vi "Write device.vi"(8 "error in (no error)":errorcluster, 10 "device":string, 11 "Update Ctl Device Setpoint MSG in":refnum<class "Update Ctl Device Setpoint MSG.lvclass">) -> (0 "error out":errorcluster, 3 "Update Ctl Device Setpoint MSG out":refnum<class "Update Ctl Device Setpoint MSG.lvclass">)   [LabVIEW 2016, in "Controller.lvlib" / "Update Ctl Device Setpoint MSG.lvclass"]
uses:
  Update Ctl Device Setpoint MSG.lvclass
  Update Ctl Device Setpoint MSG.lvclass/Update Ctl Device Setpoint MSG.ctl
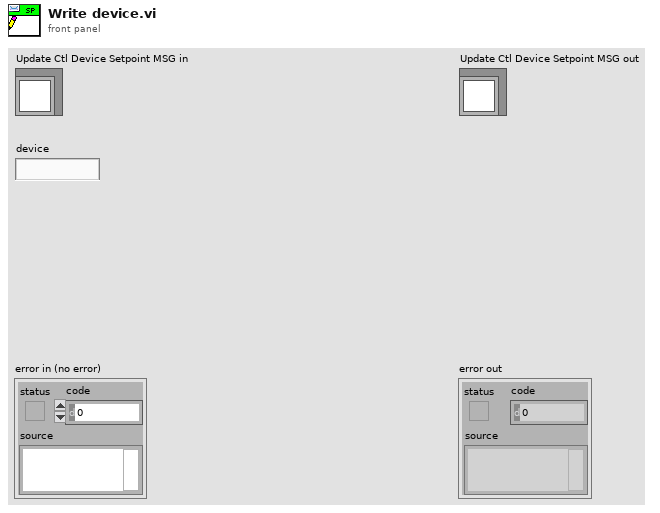
[diagram p1: front panel]
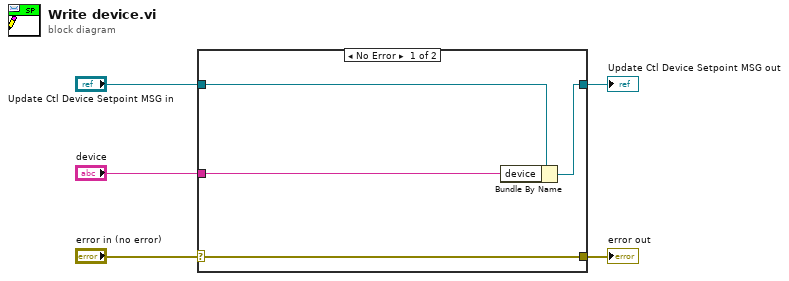
[diagram p0: block diagram]
diagram:
  n1 = case shown="No Error" "error in (no error)" {
    selector: "error in (no error)" -> [w9 w10]
    tunnel: [w9 w10] -> w4
    tunnel: [w7 w11] -> w2
    tunnel: "Update Ctl Device Setpoint MSG in" -> [w8 w11]
    tunnel: "device" -> [w6 _]
    frame No Error {
      n2 = Bundle By Name(cluster=w8, "device"=w6) -> (w7:refnum<class "Update Ctl Device Setpoint MSG.lvclass">)
    }
    frame Error {
    }
  }
  "error out" <- w4
  "Update Ctl Device Setpoint MSG out" <- w2
